vi "validate configuration.vi"(8 "error in":errorcluster, 11 "Standard Engine Repo Data in":refnum<class "synchronous engine configuration.lvclass">) -> (0 "error out":errorcluster, 3 "Standard Engine Repo Data out":refnum<class "synchronous engine configuration.lvclass">)   [LabVIEW 2013, in "synchronous engine configuration.lvclass"]
uses:
  synchronous engine configuration.lvclass
  Engine Configuration/engine configuration.lvclass
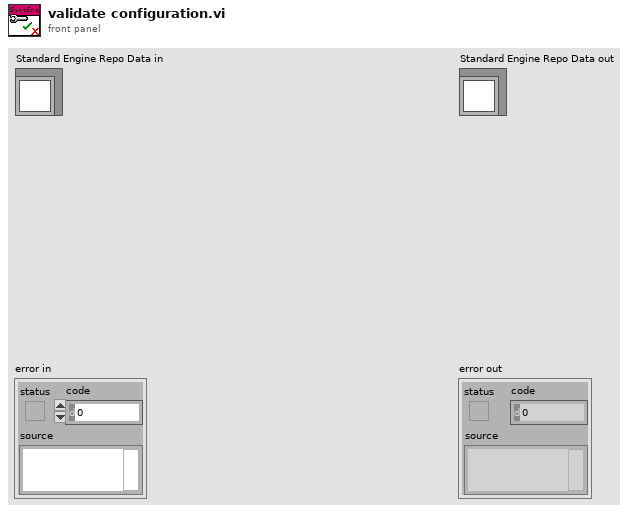
[diagram p1: front panel]
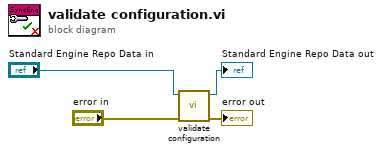
[diagram p0: block diagram]
diagram:
  n1 = call-parent "validate configuration.vi"("error in"="error in", "engine configuration in"="Standard Engine Repo Data in") -> ("error out"=→"error out":errorcluster, "engine configuration out"=→"Standard Engine Repo Data out":refnum<class "synchronous engine configuration.lvclass">)  [unwired: 8 in]
